vi "_Get Interface.vi"(2 "Desired Interface":refnum<class "IUnknown.lvclass">, 3 "Interfaceable in":refnum<class "Interfaceable.lvclass">, 4 "Available Concrete Interfaces":refnum<class "IUnknown.lvclass">[](array[class]), 9 "error in (no error)":errorcluster) -> (0 "Concrete Interface":refnum<class "IUnknown.lvclass">, 6 "error out":errorcluster)   [LabVIEW 2009, in "Interfaceable.lvclass"]
doc: "Returns a specific concrete interface from an array of concrete interfaces and injects the interfaceable object into the concrete interface."
uses:
  Interfaceable.lvclass
  IUnknown Class/IUnknown.lvclass
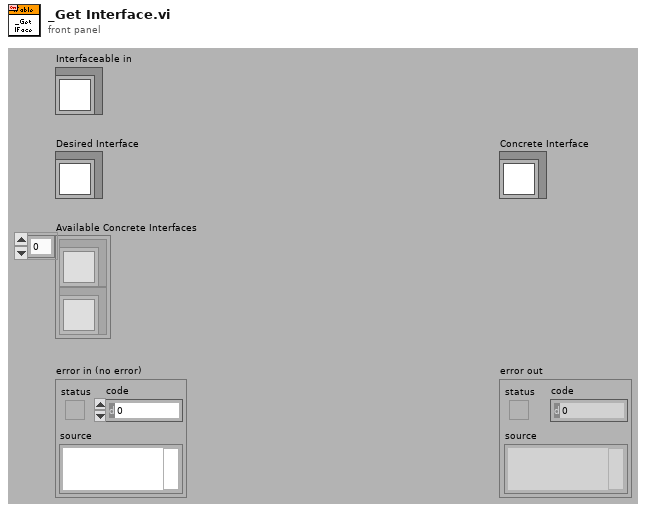
[diagram p1: front panel]
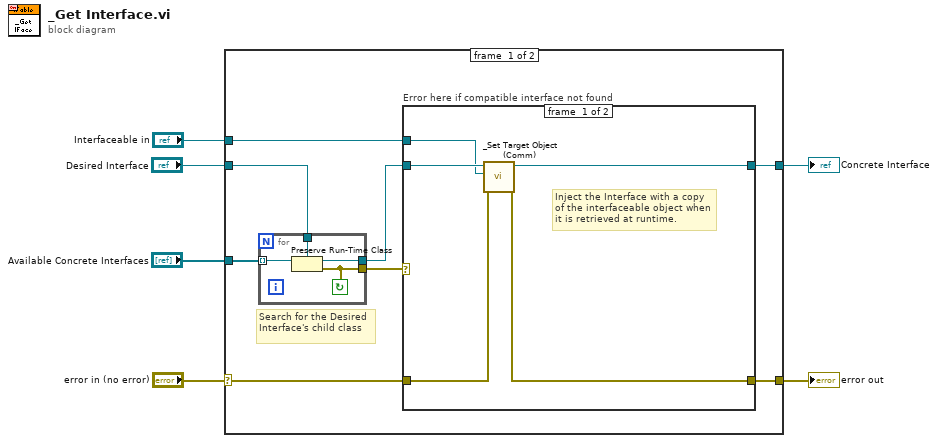
[diagram p0: block diagram]
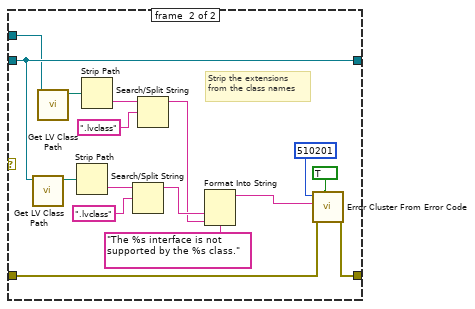
[diagram p2: hidden frame]
diagram:
  n1 = case shown="No Error" "error in (no error)" {
    selector: "error in (no error)" -> [w7 w41]
    tunnel: [w12 w41] -> w5
    tunnel: "Interfaceable in" -> [w13 _]
    tunnel: [w14 w40] -> w3
    tunnel: "Available Concrete Interfaces" -> [w10 _]
    tunnel: "Desired Interface" -> [w11 w40]
    frame #0 {
      # "Search for the Desired Interface's child class"
      n2 = for {
        tunnel: w10 -> [w38] mode=indexing
        tunnel: [w39] -> w9
        tunnel: [w37] -> w8
        tunnel: w11 -> [w36]
        stop <- w37 continue-if-true
        n3 = Preserve Run-Time Class(object in=w38, 2:w36) -> (object out=w39:refnum<class "IUnknown.lvclass">, error out=w37:errorcluster)  [unwired: 1 in]
      }
      n4 = case "Error here if compatible interface not found" shown="Error" w8 {
        tunnel: [w19 w30] -> w14
        tunnel: w13 -> [w15 w21]
        tunnel: [w18 w29] -> w12
        tunnel: w9 -> [w17 w30]
        tunnel: w7 -> [w16 w28]
        frame #0 {
          # "Inject the Interface with a copy of the interfaceable object when it is retrieved at runtime."
          n5 = call "_Set Target Object (Comm).vi"("error in (no error)"=w16, "Target Object"=w15, "Interface in"=w17) -> ("error out"=w18:errorcluster, "Interface out"=w19:refnum<class "IUnknown.lvclass">)  [unwired: 7 in]
        }
        frame #1 {
          # "Strip the extensions from the class names"
          n6 = call <vilib>:"Get LV Class Path.vi"("object"=w30) -> ("class path"=w32:path)  [unwired: 9 in, 1 out]
          n7 = call <vilib>:"Get LV Class Path.vi"("object"=w21) -> ("class path"=w22:path)  [unwired: 9 in, 1 out]
          n8 = Strip Path(path=w32) -> (name=w27:string)  [unwired: 1 out]
          n9 = Strip Path(path=w22) -> (name=w23:string)  [unwired: 1 out]
          n10 = Search/Split String(string=w27, search string/char (-)=".lvclass") -> (substring before match=w25:string)  [unwired: 1 in, 2 out]
          n11 = Search/Split String(string=w23, search string/char (-)=".lvclass") -> (substring before match=w20:string)  [unwired: 1 in, 2 out]
          n12 = Format Into String(format string="The %s interface is not supported by the %s class.", w25, w20) -> (resulting string=w34:string)  [unwired: 2 in, 1 out]
          n13 = call <vilib>:"Error Cluster From Error Code.vi"("show call chain? (False)"=TRUE, "error in (no error)"=w28, "error message (\"\")"=w34, "error code (0)"=510201) -> ("error out"=w29:errorcluster)  [unwired: 5 in]
        }
      }
    }
    frame #1 {
    }
  }
  "error out" <- w5
  "Concrete Interface" <- w3
